vi "MDC_moving.vi"(3 "Error in":errorcluster) -> (0 "Error out":errorcluster, 2 "moving?":bool)   [LabVIEW 2017]
doc: "This vi delivers the current moving status"
uses:
  HoppingSICM_v1/DLLs/MMC.dll
panel:
  # "MDC_moving"
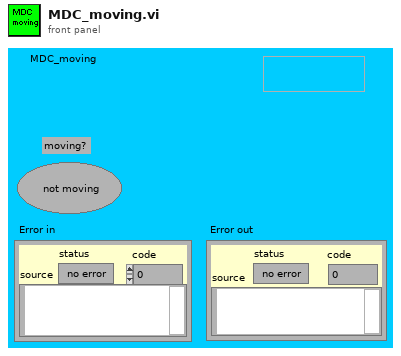
[diagram p1: front panel]
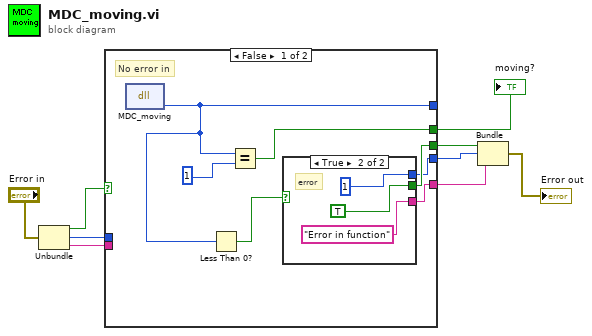
[diagram p0: block diagram]
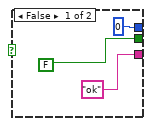
[diagram p2: hidden frame]
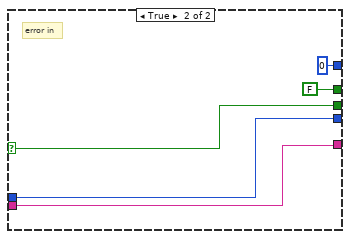
[diagram p3: hidden frame]
diagram:
  n1 = Unbundle("Error in") -> ("status"=w5:bool, "code"=w3:i32, "source"=w4:string)
  n2 = case shown="False" w5 {
    selector: w5 -> [_ w25]
    tunnel: [w14 w26] -> w9
    tunnel: [w15 w25] -> w8
    tunnel: [w16 w27] -> w7
    tunnel: w4 -> [_ w27]
    tunnel: w3 -> [_ w26]
    tunnel: [w12 0] -> _
    tunnel: [w10 FALSE] -> w2
    frame False {
      # "No error in"
      n3 = dll-call lib="F:/programmings/HoppingSICM_v1/DLLs/MMC.dll" fn="MDC_moving"() -> (w12:i32)  [unwired: 3 in, 2 out]
      n4 = Less Than 0?(x=w12) -> (x < 0?=w11:bool)
      n5 = Equal?(x=w12, y=1) -> (x = y?=w10:bool)
      n6 = case shown="True" w11 {
        tunnel: ["ok" "Error in function"] -> w16
        tunnel: [FALSE TRUE] -> w15
        tunnel: [0 1] -> w14
        frame False {
        }
        frame True {
          # "error"
        }
      }
    }
    frame True {
      # "error in"
    }
  }
  "moving?" <- w2
  n7 = Bundle(w8, "code"=w9, "source"=w7) -> (→"Error out":cluster{bool, "code":i32, "source":string})  [unwired: 1 in]
